vi "Initialize.vi"(8 "error in (no error)":errorcluster, 9 "Build Configurations":string[](array[string]), 10 "Preceding Items":refnum<class "Item.lvclass">[](array[class]), 11 "Build Package Item in":refnum<class "VIPM Item.lvclass">) -> (0 "error out":errorcluster, 3 "Item out":refnum<class "Item.lvclass">)   [LabVIEW 2019, in "VIPM.lvlib" / "VIPM Item.lvclass"]
uses:
  VIPM Item.lvclass
  C:/Users/pasca/source/repos/mgi-solution-explorer-extensions/libs/Solution.lvlibp/Solution/Item/Item.lvclass
  libs/Solution.lvlibp/Solution/Item/Item.lvclass
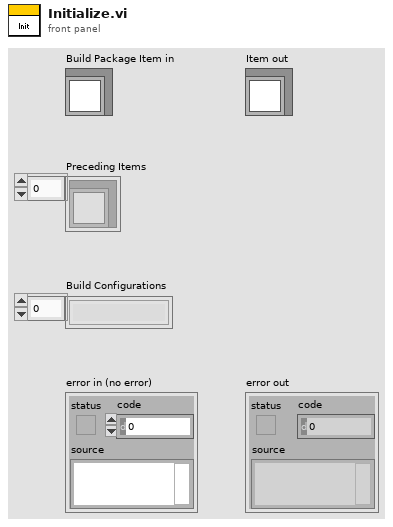
[diagram p1: front panel]
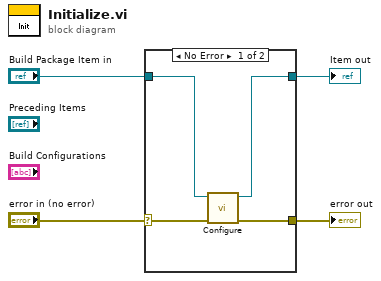
[diagram p0: block diagram]
diagram:
  n1 = case shown="No Error" "error in (no error)" {
    selector: "error in (no error)" -> [w8 w9]
    tunnel: [w7 w9] -> w3
    tunnel: "Build Package Item in" -> [w6 w10]
    tunnel: [w5 w10] -> w1
    frame No Error {
      n2 = call "Configure.vi"("error in (no error)"=w8, "Build Package Item in"=w6) -> ("error out"=w7:errorcluster, "Build Package Item out"=w5:refnum<class "VIPM Item.lvclass">)  [unwired: 8 in]
    }
    frame Error {
    }
  }
  "error out" <- w3
  "Item out" <- w1
